vi "Relation Definition.vi"(11 "Relation in":refnum<class "Relation.lvclass">) -> (1 "Relation Definition":T1={"Mapping"=enum."OneToMany", "Related To"="", "Reversed By"="", "Related Class"=""}, 2 "Table Name":string, 3 "Relation out":refnum<class "Relation.lvclass">)   [LabVIEW 2020, in "Conditu2.lvlib" / "Columns.lvlib" / "Relation.lvclass"]
uses:
  Relation.lvclass
  C:/dev/lv20CE/lv-conditum-tools/Conditum-Clone/Columns/Type/Type.lvclass
  Relation Info.ctl
  Relation Mapping.ctl
  Type/Type.lvclass/Type.ctl
  Relation.lvclass/Relation.ctl
  Type/Type.lvclass
  Conditu2.lvlib
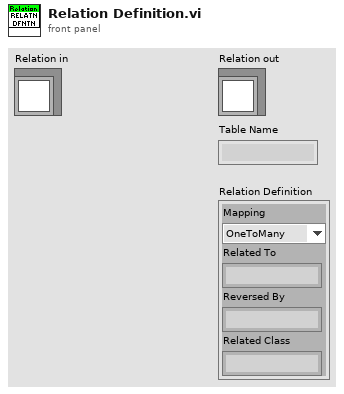
[diagram p1: front panel]
types:
  T1 = typedef "Conditu2.lvlib/Relation Info.ctl" = cluster{"Mapping":T2, "Related To":string, "Reversed By":string, "Related Class":string}
  T2 = typedef "Conditu2.lvlib/Relation Mapping.ctl" = enum16{"OneToOne", "OneToMany", "ManyToOne", "ManyToMany"}
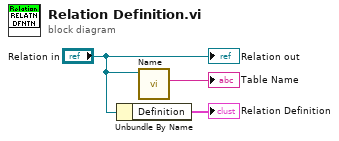
[diagram p0: block diagram]
diagram:
  n1 = Unbundle By Name("Relation in") -> ("Definition"=→"Relation Definition":T1)
  n2 = call "Name.vi"("Type in"="Relation in") -> ("Table Name"=→"Table Name":string)  [unwired: 10 in]
  "Relation out" <- "Relation in"
